vi "MV3D RGBD YUV422To RGB.vi"(10 "pRgbImage":T1, 11 "pYuvImgge":T1) -> (1 "function return":i32, 2 "pRgbImage out":T1, 3 "pYuvImgge out":T1)   [LabVIEW 2015, in "Mv3dRgbdEx.lvlib"]
doc: "MV3D_RGBD_API_Ex MV3D_RGBD_STATUS MV3D_RGBD_YUV422ToRGB(MV3D_RGBD_IMAGE_DATA *pYuvImgge, MV3D_RGBD_IMAGE_DATA* pRgbImage);"
uses:
  <userlib>/Mv3dRgbdEx/Mv3dRgbdEx.lvlib
  <userlib>/Mv3dRgbdEx/Mv3dRgbdEx.dll
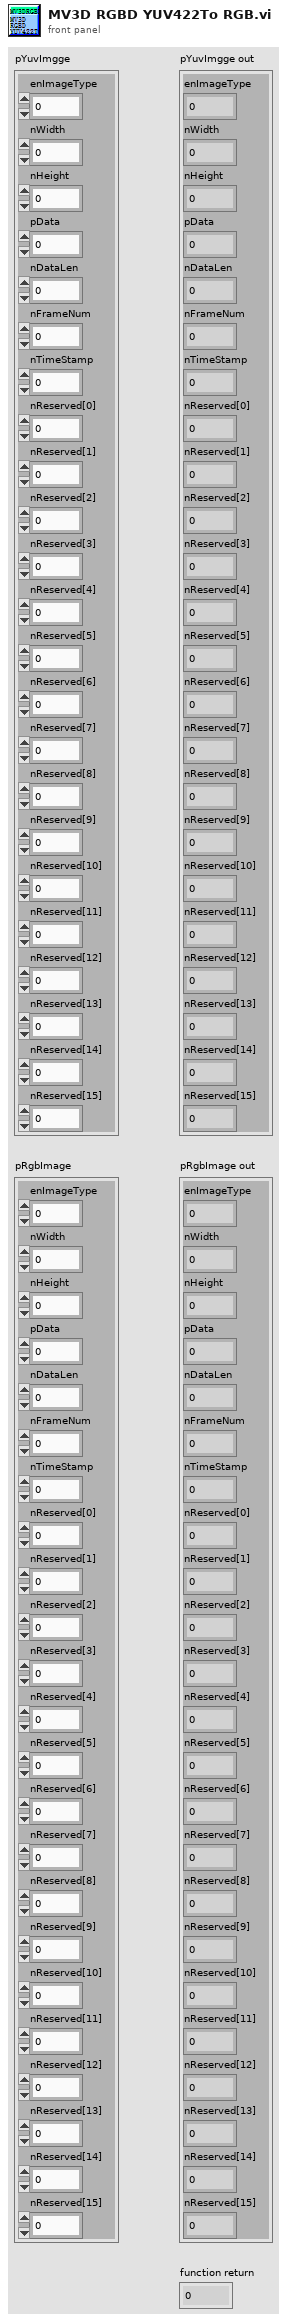
[diagram p1: front panel]
types:
  T1 = cluster{"enImageType":i32, "nWidth":u32, "nHeight":u32, "pData":u32, "nDataLen":u32, "nFrameNum":u32, "nTimeStamp":i64, "nReserved[0]":u8, "nReserved[1]":u8, "nReserved[2]":u8, "nReserved[3]":u8, "nReserved[4]":u8, "nReserved[5]":u8, "nReserved[6]":u8, "nReserved[7]":u8, "nReserved[8]":u8, "nReserved[9]":u8, "nReserved[10]":u8, "nReserved[11]":u8, "nReserved[12]":u8, "nReserved[13]":u8, "nReserved[14]":u8, "nReserved[15]":u8}
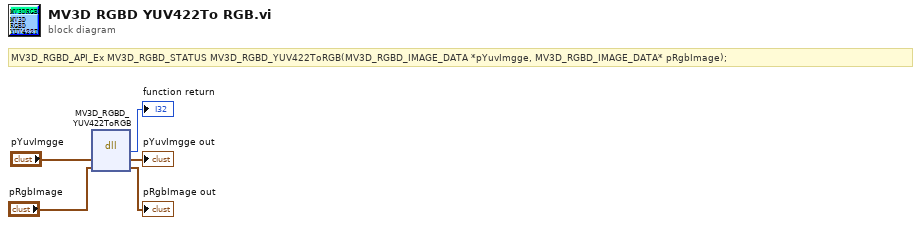
[diagram p0: block diagram]
diagram:
  # "MV3D_RGBD_API_Ex MV3D_RGBD_STATUS MV3D_RGBD_YUV422ToRGB(MV3D_RGBD_IMAGE_DATA *pYuvImgge, MV3D_RGBD_IMAGE_DATA* pRgbImage);"
  n1 = dll-call lib="C:/Program Files (x86)/National Instruments/LabVIEW 2015/user.lib/Mv3dRgbdEx/Mv3dRgbdEx.*" fn="MV3D_RGBD_YUV422ToRGB"("pYuvImgge"="pYuvImgge", "pRgbImage"="pRgbImage") -> (→"function return":i32, "pYuvImgge"=→"pYuvImgge out":T1, "pRgbImage"=→"pRgbImage out":T1)  [unwired: 3 in, 2 out]
